vi "Obtain model queue.vi"(8 "error in (no error)":errorcluster) -> (0 "error out":errorcluster, 3 "Model loop queue":refnum<queue>)   [LabVIEW 2018]
doc: "Gets a reference to the queue used by the controller.\n\nThis reference should never be destroyed. Also, as a general note, this VI shouldn't be accessed directly in most cases; it should be wrapped by other VIs to perform specific functions."
uses:
  Model queue data.ctl
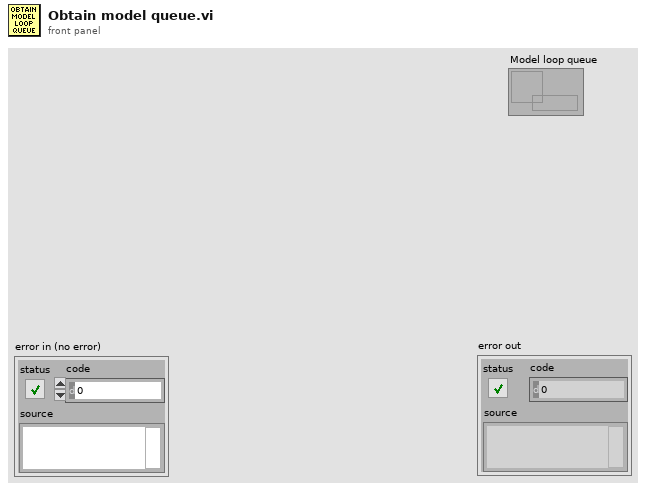
[diagram p1: front panel]
types:
  T1 = typedef "Model queue data.ctl" = cluster{"State":string, "Data":variant, "Next state if error":string}
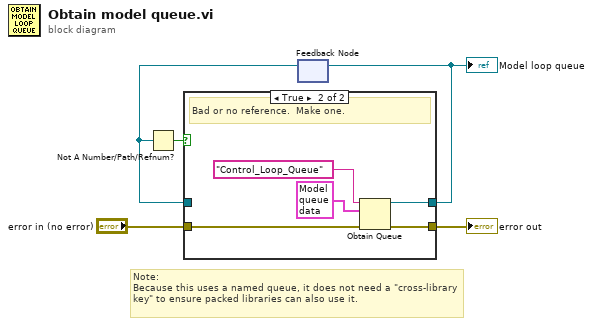
[diagram p0: block diagram]
diagram:
  # "Note:\nBecause this uses a named queue, it does not need a \"cross-library key\" to ensure packed libraries can also use it."
  n1 = feedback #1() -> (w1:refnum<queue>)  [unwired: 1 in]
  n2 = Not A Number/Path/Refnum?(number/path/refnum=w1) -> (NaN/Path/Refnum?=w4:bool)
  n3 = case shown="True" w4 {
    tunnel: "error in (no error)" -> [w6 w12]
    tunnel: [w6 w11] -> w3
    tunnel: [w7 w8] -> w2
    tunnel: w1 -> [w7 _]
    frame False {
      # "Good reference last time.  Pass it out again."
    }
    frame True {
      # "Bad or no reference.  Make one."
      n4 = Obtain Queue(name (unnamed)="Control_Loop_Queue", element data type=T1 {"State"="", "Data"=variant, "Next state if error"=""} ("Control loop queue data"), error in (no error)=w12) -> (queue out=w8:refnum<queue>, error out=w11:errorcluster)  [unwired: 2 in, 1 out]
    }
  }
  "error out" <- w3
  "Model loop queue" <- w2
  n5 = feedback-in #1(w2) -> ()
